vi "FRCts20_WebMethods_ESP_TeamArray.vi"(8 "error in (no error)":errorcluster, 9 "Teams":T1, 10 "Return Type":T4="mobile", 11 "httpRequestID":u32) -> (0 "error out":errorcluster, 3 "httpRequestID out":u32)   [LabVIEW 2014, in "FRCts20_WebMethods.lvlib"]
uses:
  FRCts20_WebMethods.lvlib
  Controls/FRCts20_WebMethods_ctl_returntype.ctl
  Backend/source/VI Source/FRCts20_Backend_API/FRCts20_Backend_API_SW.ctl
  Backend/source/VI Source/FRCts20_Backend_API/FRCts20_Backend_API_Status.ctl
  Controls/FRCts20_WebMethods_ctl_teamarray.ctl
  Controls/FRCts20_WebMethods_Globals.vi
  <vilib>/wsapi/subVIs/Set String ESP Variable.vi
  <vilib>/wsapi/subVIs/Set Integer ESP Variable.vi
  Backend/source/VI Source/FRCts20_Backend_API/FRCts20_Backend_API.lvlib
  <vilib>/wsapi/NI_WebServices.lvlib
  Backend/source/VI Source/FRCts20_Backend_API/FRCts20_Backend_API_Command_Competition.ctl
  Backend/source/VI Source/FRCts20_Backend_API/FRCts20_Backend_API_Competition.ctl
  Backend/source/VI Source/INI_Accessor/FRCts20_Backend_INI Controller.lvclass
  Backend/source/VI Source/FRCts20_Backend_API/FRCts20_Backend_API_Event.vi
panel:
  in  "Status (hidden)":T2
  in  "SWType (hidden)":T3
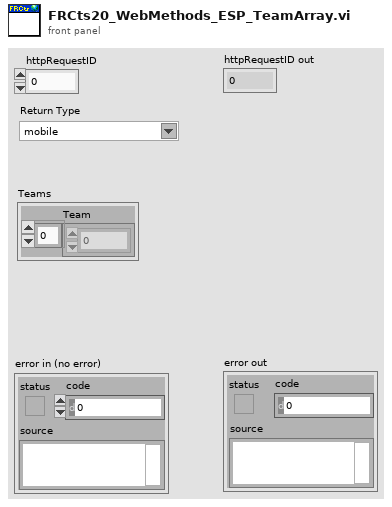
[diagram p1: front panel]
types:
  T1 = typedef "FRCts20_WebMethods.lvlib/FRCts20_WebMethods_ctl_teamarray.ctl" = cluster{"Team":u32[]}
  T2 = typedef "FRCts20_Backend_API.lvlib/FRCts20_Backend_API_Status.ctl" = enum16{"Open", "In Work", "Closed"}
  T3 = typedef "FRCts20_Backend_API.lvlib/FRCts20_Backend_API_SW.ctl" = string
  T4 = typedef "FRCts20_WebMethods.lvlib/FRCts20_WebMethods_ctl_returntype.ctl" = string
  T5 = typedef "FRCts20_Backend_API.lvlib/FRCts20_Backend_API_Competition.ctl" = cluster{"Name":string, "Start Date":timestamp, "Duration":u8, "Divisions":string[], "APIReturn":string}
  T6 = typedef "FRCts20_Backend_API.lvlib/FRCts20_Backend_API_Command_Competition.ctl" = string
  T7 = typedef "FRCts20_Backend_API.lvlib/FRCts20_Backend_API_Event.ctl" = cluster{"Event Index":u32, "Name":string, "Start Time":timestamp, "End Time":timestamp, "Teams":cluster{"Team Index":u32, "Team Number":u32, "Requests":cluster{"Request Number":u32, "Description":string}[], "Has Open Issue":bool}[], "SWType":T3, "APIReturn":string}
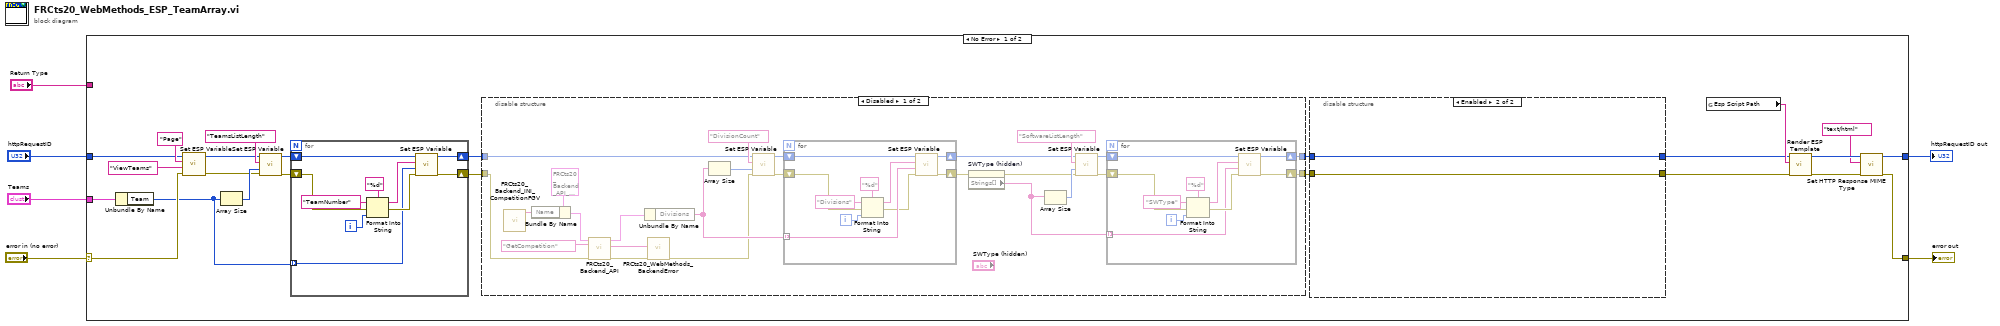
[diagram p0: block diagram]
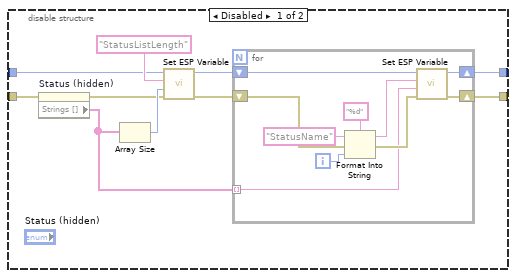
[diagram p2: hidden frame]
diagram:
  n1 = case shown="No Error" "error in (no error)" {
    selector: "error in (no error)" -> [w14 w111]
    tunnel: "httpRequestID" -> [w17 w110]
    tunnel: [w28 w110] -> w3
    tunnel: [w27 w111] -> w2
    tunnel: "Return Type" -> [_ _]
    tunnel: "Teams" -> [w20 _]
    frame No Error {
      n2 = Unbundle By Name(w20) -> ("Team"=w13:u32[])
      n3 = call-poly <vilib>:"Set ESP Variable.vi"("error in (no error)"=w14, "value"="ViewTeams", "key"="Page", "httpRequestID"=w17) -> ("error out"=w16:errorcluster, "httpRequestID out"=w15:u32)  [unwired: 6 in]
      n4 = Array Size(array=w13) -> (size(s)=w24:i32)
      n5 = call-poly <vilib>:"Set ESP Variable.vi"("error in (no error)"=w16, "value"=w24, "key"="TeamsListLength", "httpRequestID"=w15) -> ("error out"=w22:errorcluster, "httpRequestID out"=w21:u32)  [unwired: 6 in]
      n6 = for {
        shift-right: [w101] -> w11
        shift-left: w22 -> [w104]
        shift-right: [w100] -> w12
        shift-left: w21 -> [w109]
        tunnel: w13 -> [w102] mode=indexing
        i -> [w105]
        n7 = Format Into String(format string="%d", initial string="TeamNumber", error in=w104, w105) -> (resulting string=w107:string, error out=w103:errorcluster)
        n8 = call-poly <vilib>:"Set ESP Variable.vi"("error in (no error)"=w103, "value"=w102, "key"=w107, "httpRequestID"=w109) -> ("error out"=w101:errorcluster, "httpRequestID out"=w100:u32)  [unwired: 6 in]
      }
      n9 = disable-structure shown="Disabled" {
        disable-tunnel: w12 -> [w70 w99]
        disable-tunnel: w11 -> [w69 w98]
        disable-tunnel: [w59 w99] -> w10
        disable-tunnel: [w56 w98] -> w7
        frame Disabled {
          n10 = call "FRCts20_Backend_INI_CompetitionFGV.vi"() -> ("Value out"=w54:string)  [unwired: 11 in]
          n11 = Bundle By Name(cluster=T5 {"Name"="", "Start Date"=timestamp(0 s since 1904-01-01), "Duration"=0, "Divisions"=[], "APIReturn"=""} ("Competition In"), "Name"=w54) -> (w53:T5)
          n12 = call-poly "FRCts20_Backend_API.vi"("error in (no error)"=w69, "Command"=T6 "GetCompetition", "Event In"=w53) -> ("error out"=w68:errorcluster, "Status"=w67:string, "Event Out"=w77:T7)  [unwired: 6 in]
          n13 = Unbundle By Name(w77) -> ("Divisions"=w74:string[])
          n14 = call "FRCts20_WebMethods_BackendError.vi"("error in (no error)"=w68, "Status"=w67) -> ("error out"=w66:errorcluster)  [unwired: 8 in, 1 out]
          n15 = Array Size(array=w74) -> (size(s)=w76:i32)
          n16 = call-poly <vilib>:"Set ESP Variable.vi"("error in (no error)"=w66, "value"=w76, "key"="DivisionCount", "httpRequestID"=w70) -> ("error out"=w73:errorcluster, "httpRequestID out"=w72:u32)  [unwired: 6 in]
          n17 = for {
            tunnel: w74 -> [w92] mode=indexing
            shift-right: [w97] -> w58
            shift-left: w73 -> [w89]
            shift-right: [w90] -> w62
            shift-left: w72 -> [w96]
            i -> [w94]
            n18 = Format Into String(format string="%d", initial string="Divisions", error in=w89, w94) -> (resulting string=w93:string, error out=w88:errorcluster)
            n19 = call-poly <vilib>:"Set ESP Variable.vi"("error in (no error)"=w88, "value"=w92, "key"=w93, "httpRequestID"=w96) -> ("error out"=w97:errorcluster, "httpRequestID out"=w90:u32)  [unwired: 6 in]
          }
          n20 = property on="SWType (hidden)" class="CmbBox (strict)"(error in=w58) -> (error out=w57:errorcluster, "Strings[]"=w60:string[])  [unwired: 1 in, 1 out]
          n21 = Array Size(array=w60) -> (size(s)=w61:i32)
          n22 = call-poly <vilib>:"Set ESP Variable.vi"("error in (no error)"=w57, "value"=w61, "key"="SoftwareListLength", "httpRequestID"=w62) -> ("error out"=w64:errorcluster, "httpRequestID out"=w65:u32)  [unwired: 6 in]
          n23 = for {
            shift-right: [w87] -> w56
            shift-left: w64 -> [w80]
            shift-right: [w81] -> w59
            shift-left: w65 -> [w86]
            tunnel: w60 -> [w78] mode=indexing
            i -> [w84]
            n24 = Format Into String(format string="%d", initial string="SWType", error in=w80, w84) -> (resulting string=w83:string, error out=w79:errorcluster)
            n25 = call-poly <vilib>:"Set ESP Variable.vi"("error in (no error)"=w79, "value"=w78, "key"=w83, "httpRequestID"=w86) -> ("error out"=w87:errorcluster, "httpRequestID out"=w81:u32)  [unwired: 6 in]
          }
        }
        frame Enabled {
        }
      }
      n26 = disable-structure shown="Enabled" {
        disable-tunnel: w10 -> [w37 w52]
        disable-tunnel: [w36 w51] -> w9
        disable-tunnel: [w35 w52] -> w8
        disable-tunnel: w7 -> [w34 w51]
        frame Disabled {
          n27 = property on="Status (hidden)" class="Enum (strict)"(error in=w34) -> (error out=w31:errorcluster, "Strings []"=w32:string[])  [unwired: 1 in, 1 out]
          n28 = Array Size(array=w32) -> (size(s)=w33:i32)
          n29 = call-poly <vilib>:"Set ESP Variable.vi"("error in (no error)"=w31, "value"=w33, "key"="StatusListLength", "httpRequestID"=w37) -> ("error out"=w39:errorcluster, "httpRequestID out"=w38:u32)  [unwired: 6 in]
          n30 = for {
            shift-right: [w50] -> w36
            shift-left: w39 -> [w43]
            shift-right: [w44] -> w35
            shift-left: w38 -> [w49]
            tunnel: w32 -> [w41] mode=indexing
            i -> [w47]
            n31 = Format Into String(format string="%d", initial string="StatusName", error in=w43, w47) -> (resulting string=w46:string, error out=w42:errorcluster)
            n32 = call-poly <vilib>:"Set ESP Variable.vi"("error in (no error)"=w42, "value"=w41, "key"=w46, "httpRequestID"=w49) -> ("error out"=w50:errorcluster, "httpRequestID out"=w44:u32)  [unwired: 6 in]
          }
        }
        frame Enabled {
        }
      }
      n33 = global read "FRCts20_WebMethods_Globals.vi" "Esp Script Path"() -> (w26:string)
      n34 = call <vilib>:"Render ESP Template.vi"("error in (no error)"=w9, "espName"=w26, "httpRequestID"=w8) -> ("error out"=w29:errorcluster, "httpRequestID out"=w30:u32)  [unwired: 7 in]
      n35 = call <vilib>:"Set HTTP Response MIME Type.vi"("error in (no error)"=w29, "MIME type (text/html)"="text/html", "httpRequestID"=w30) -> ("error out"=w27:errorcluster, "httpRequestID out"=w28:u32)  [unwired: 7 in]
    }
    frame Error {
    }
  }
  "httpRequestID out" <- w3
  "error out" <- w2
